vi "destroy UI user event.vi"(11 "Template in":refnum<class "Template.lvclass">) -> (0 "error out":errorcluster)   [LabVIEW 2020, in "Template.lvlib" / "Template.lvclass"]
uses:
  Template.lvclass
  Template.lvclass/Template.ctl
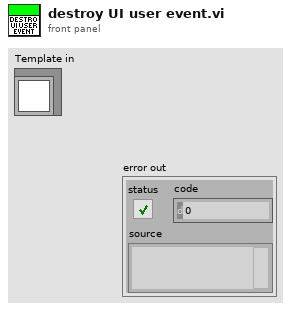
[diagram p1: front panel]
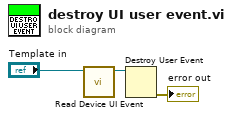
[diagram p0: block diagram]
diagram:
  n1 = call "Read Device UI Event.vi"("Template in"="Template in") -> ("Device UI Event"=w2:refnum<user-event>)  [unwired: 10 in]
  n2 = Destroy User Event(user event=w2) -> (error out=→"error out":errorcluster)  [unwired: 1 in]
